vi "Lookup Devices by Type.vi"(8 "error in (no error)":errorcluster, 10 "Hardware Type":string, 11 "Controller in":refnum<class "Controller.lvclass">) -> (0 "error out":errorcluster, 2 "Matching Devices":string[](array[string]), 3 "Controller out":refnum<class "Controller.lvclass">)   [LabVIEW 2016, in "Controller Actor.lvlib" / "Controller.lvclass"]
uses:
  <userlib>/Common Components/Controller/Controller.lvclass
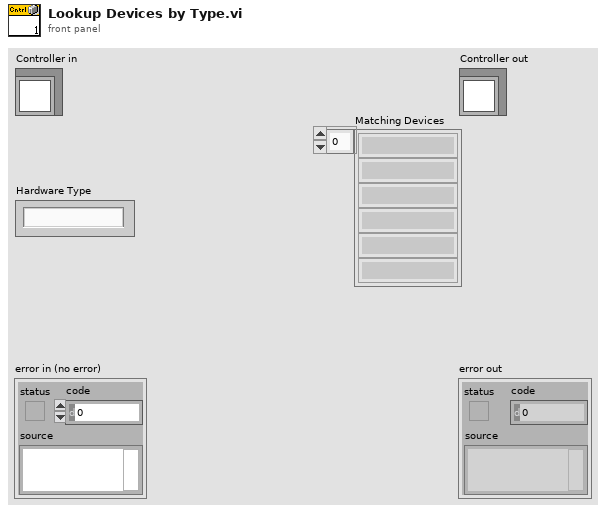
[diagram p1: front panel]
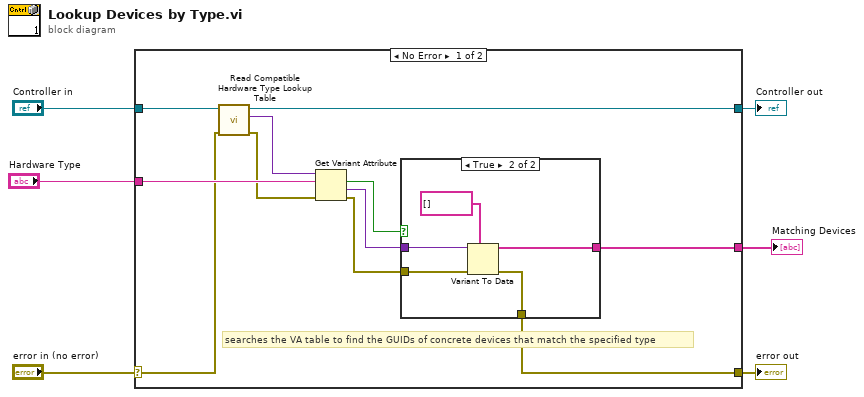
[diagram p0: block diagram]
diagram:
  n1 = case shown="No Error" "error in (no error)" {
    selector: "error in (no error)" -> [w9 w25]
    tunnel: [w8 w25] -> w5
    tunnel: [w12 w24] -> w3
    tunnel: "Controller in" -> [w17 w24]
    tunnel: "Hardware Type" -> [w15 _]
    tunnel: [w13 _] -> w1
    frame No Error {
      # "searches the VA table to find the GUIDs of concrete devices that match the specified type"
      n2 = call <userlib>:"Read Compatible Hardware Type Lookup Table.vi"("error in (no error)"=w9, "Controller in"=w17) -> ("error out"=w10:errorcluster, "Compatible Hardware Type Lookup Table"=w16:variant, "Controller out"=w12:refnum<class "Controller.lvclass">)  [unwired: 7 in]
      n3 = Get Variant Attribute(Variant=w16, name=w15, error in=w10) -> (found=w7:bool, value=w14:variant, error out=w11:errorcluster)  [unwired: 1 in, 1 out]
      n4 = case shown="True" w7 {
        tunnel: w14 -> [_ w22]
        tunnel: [_ w21] -> w13
        tunnel: w11 -> [w18 w20]
        tunnel: [w18 w19] -> w8
        frame False {
        }
        frame True {
          n5 = Variant To Data(error in=w20, type=string[] [], Variant=w22) -> (data=w21:string[], error out=w19:errorcluster)
        }
      }
    }
    frame Error {
    }
  }
  "error out" <- w5
  "Controller out" <- w3
  "Matching Devices" <- w1
